vi "TcpIDFGV.vi"(8 "Error In":errorcluster, 10 "action":enum16{"write", "read"}(ring), 11 "connection ID in":refnum<k5>) -> (0 "Error Out":errorcluster, 3 "connection ID out":refnum<k5>)   [LabVIEW 2020]
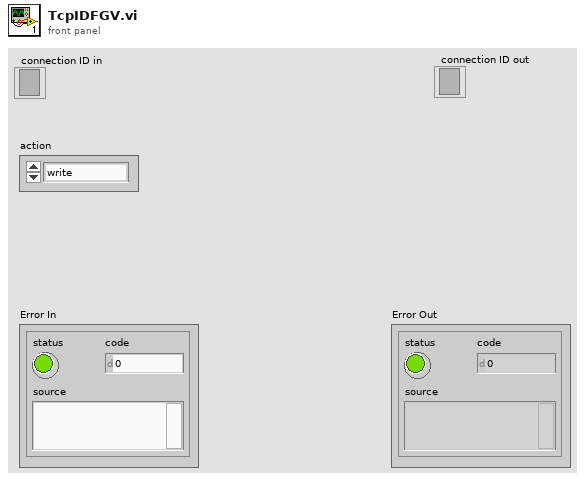
[diagram p1: front panel]
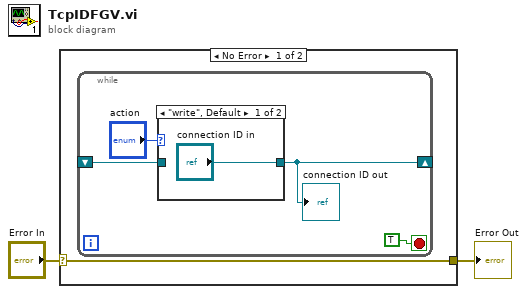
[diagram p0: block diagram]
diagram:
  n1 = case shown="No Error" "Error In" {
    selector: "Error In" -> [w3 w10]
    tunnel: [w3 w10] -> w1
    frame No Error {
      n2 = while {
        shift-right: [w5] -> _
        shift-left: _ -> [w4]
        stop <- TRUE stop-if-true
        n3 = case shown="\"write\", Default" "action" {
          tunnel: ["connection ID in" w9] -> w5
          tunnel: w4 -> [_ w9]
          frame "write", Default {
          }
          frame "read" {
          }
        }
        "connection ID out" <- w5
      }
    }
    frame Error {
    }
  }
  "Error Out" <- w1
